vi "read_matrix_test.vi"() -> ()   [LabVIEW 2012]
uses:
  read_matrix_reshape_4D.vi
panel:
  out "output array":dbl[][][][](array[numeric])
  in  "Path":path
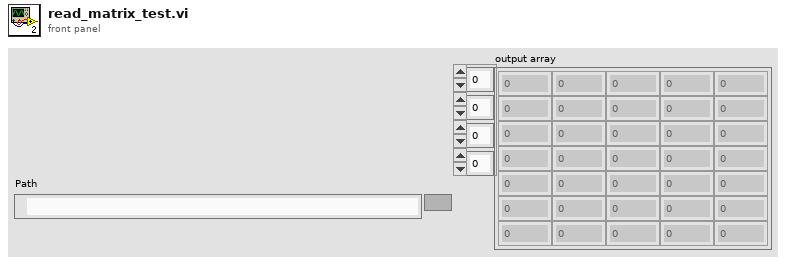
[diagram p1: front panel]
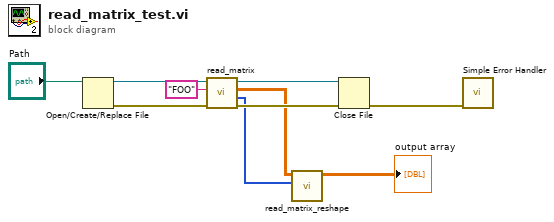
[diagram p0: block diagram]
diagram:
  n1 = Open/Create/Replace File(file path (use dialog)="Path") -> (refnum out=w9:refnum<file>, error out=w8:errorcluster)  [unwired: 5 in, 1 out]
  n2 = call "read_matrix.vi"("error in"=w8, "Entry name"="FOO", "file refnum"=w9) -> ("error out"=w7:errorcluster, "Dimensions"=w3:i32[], "Result"=w4:dbl[][], "refnum out"=w6:refnum<file>)  [unwired: 4 in, 1 out]
  n3 = call-poly "read_matrix_reshape.vi"("Dimensions"=w3, "Result in"=w4) -> ("Result out"=→"output array":dbl[][][][])  [unwired: 9 in]
  n4 = Close File(refnum=w6, error in=w7) -> (error out=w5:errorcluster)  [unwired: 1 out]
  n5 = call <vilib>:"Simple Error Handler.vi"("error in (no error)"=w5) -> ()  [unwired: 4 in, 5 out]
